vi "Calibrate White Balancev1.vi"() -> ()   [LabVIEW 2013]
uses:
  <vilib>/Rock Robotics/WPI/Camera/WPI_CameraWhite Balance Values.ctl
panel:
  out "Camera Image":T1(plugin-control)
  in  "stop":bool
  # "Instructions for calibrating white balance:\n1. Run this VI.\n2. Hold finger over the camera lens for ~5 seconds.\n     This empties the camera WB history, causing it to adapt more quickly when exposed to light.\n3. Remove finger and point camera at a scene that contains something white (copier paper several feet from camera works well).\n     This lets the camera adapt to the current lighting reflected from the white paper.    \n4. Click the stop button.\n     The camera is now set to use and remember this white balance setting until you change it.\n\nRationale:\nAutomatic white balance continually updates the camera sensor's color processing gains to make near white objects more white by\nsubtracting their tint from the entire scene. Normally this is a good thing, neutralizing the yellow tint of incandescent bulbs, or the\nblue-green tint of fluorescents as they reflect from whatever white object is in the scene.\n\nUnfortunately, when given a typical FRC scene with a brightly colored objects, the same white balance algorithm may attempt to\nturn one of the bright objects white instead. It will subtract more and more of the target color over time until the brightly colored\ntarget is no longer brightly colored. Left exposed to the scene for even a few minutes, the algorithm may misinterpret and adapt poorly,\ndefeating your color based measurements. For this reason, we recommend calibrating using this algorithm in light reasonably close to\nwhat the robot will be expected to operate in, then set the camera to hold the settings.\n\nFor repeatable results, pay attention to the white object used for calibration, the angle of this object to the lighting, and the distance\nfrom the camera lens. It should not be necessary to recalibrate unless the lighting changes significantly. A good indicator is when a known\ntarget's color no longer matches the color thresholds previously used for identification."
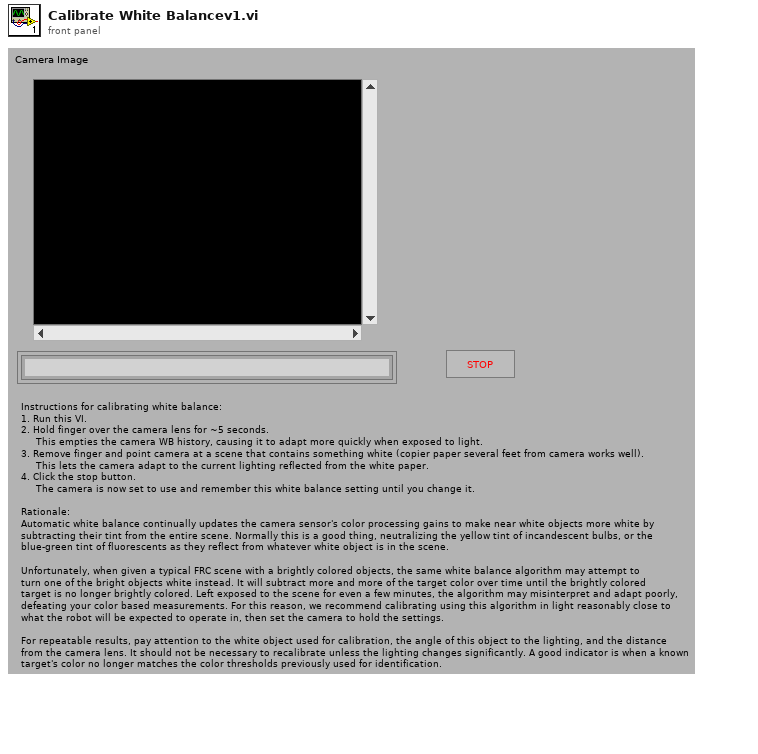
[diagram p1: front panel]
types:
  T1 = typedef "IMAQ Image.ctl" = refnum<image>
  T2 = typedef "Image Type" = u32
  T3 = typedef "WPI_CameraWhite Balance Values.ctl" = enum16{"Auto", "Fixed indoor", "Fixed outdoor 1", "Fixed outdoor 2", "Fixed fluorescent 1", "Fixed fluorescent 2", "Hold current"}
  T4 = typedef "WPI_CameraDevRef.ctl" = cluster{"Camera Address":string, "CameraStatus":errorcluster, "Acquire Image Notifier":refnum<notifier>}
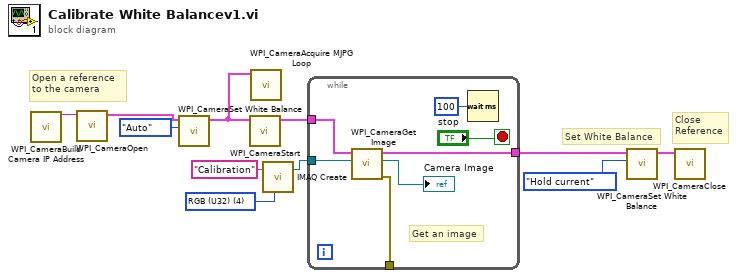
[diagram p0: block diagram]
diagram:
  w6 = T2 4 items=["Grayscale (U8)", "Grayscale (I16)", "Grayscale (SGL)", "Complex (CSG)", "RGB (U32)", "HSL (U32)", "RGB (U64)", "Grayscale (U16)"] ("Image Type")
  # "Close\nReference"
  # "Set White Balance"
  # "Open a reference \nto the camera"
  n1 = call <vilib>:"WPI_CameraBuild Camera IP Address.vi"() -> ("Camera Address"=w1:string)  [unwired: 11 in]
  n2 = call <vilib>:"WPI_CameraOpen.vi"("Camera Address"=w1) -> ("CameraDevRef"=w8:T4)  [unwired: 1 in, 9 out]
  n3 = call <vilib>:"WPI_CameraSet White Balance.vi"("White Balance"=WPI_CameraWhite_Balance_Values."Auto", "CameraDevRef"=w8) -> ("CameraDevRef Out"=w3:T4)  [unwired: 1 in, 8 out]
  n4 = call <vilib>:"WPI_CameraStart.vi"("CameraDevRef"=w3) -> ("CameraDevRef Out"=w4:T4)  [unwired: 1 in, 9 out]
  n5 = call <vilib>:"WPI_CameraAcquire MJPG Loop.vi"("CameraDevRef"=w3) -> ()  [unwired: 11 in]
  n6 = call "IMAQ Create"("Image Name"="Calibration", "Image Type"=w6) -> ("New Image"=w5:T1)  [unwired: 2 in, 2 out]
  n7 = while {
    tunnel: [w15] -> w11
    tunnel: w4 -> [w16]
    tunnel: w5 -> [w14]
    tunnel: [w12] -> _
    stop <- "stop" stop-if-true
    # "Get an image"
    n8 = call <vilib>:"WPI_CameraGet Image.vi"("Image"=w14, "CameraDevRef"=w16) -> ("error out"=w12:errorcluster, "Image Out"=→"Camera Image":T1, "CameraDevRef Out"=w15:T4)  [unwired: 1 in, 6 out]
    n9 = Wait (ms)(milliseconds to wait=u32 100) -> ()  [unwired: 1 out]
  }
  n10 = call <vilib>:"WPI_CameraSet White Balance.vi"("White Balance"=WPI_CameraWhite_Balance_Values."Hold current", "CameraDevRef"=w11) -> ("CameraDevRef Out"=w2:T4)  [unwired: 1 in, 8 out]
  n11 = call <vilib>:"WPI_CameraClose.vi"("CameraDevRef"=w2) -> ()  [unwired: 10 in, 1 out]
